vi "ExperimentCode_nodaq.vi"() -> ()   [LabVIEW 2017]
uses:
  <vilib>/Analysis/baseanly.llb/Mean (DBL).vi
  <vilib>/Instr/_visa.llb/VISA Configure Serial Port (Instr).vi
  <vilib>/express/express shared/transition.llb/Dynamic To Waveform Array.vi
  <vilib>/express/express signal manip/GetorSetDDTAttributes/Set DDT Attributes/SetT0.vi
  <vilib>/express/express shared/transition.llb/Waveform Array To Dynamic.vi
  <vilib>/express/express signal manip/GetorSetDDTAttributes/Set DDT Attributes/Set DDT Properties.xnode
  <vilib>/Analysis/NI_AALPro.lvlib
  <vilib>/Analysis/NI_AALBase.lvlib
panel:
  in  "Tab Control":enum32{"Setup ", "Experiment Controls", "Debug"}(tab)=enum."Experiment Controls"
  in  "Max Torque":dbl=21.3
  in  "Servo 1 Zero Offset":dbl
  in  "Servo 2 Zero Offset":dbl
  in  "Servo 3 Zero Offset":dbl
  in  "Servo 4 Zero Offset":dbl
  in  "Servo 5 Zero Offset":dbl
  in  "Servo 5 Torque Intercept":dbl
  in  "Servo 5 Torque Slope":dbl=1.0
  in  "Servo 5 Position Intercept":dbl
  in  "Servo 5 Position Slope":dbl=1.0
  in  "Servo 4 Torque Intercept":dbl
  in  "Servo 4 Torque Slope":dbl=1.0
  in  "Servo 4 Position Intercept":dbl
  in  "Servo 4 Position Slope":dbl=1.0
  in  "Servo 3 Torque Intercept":dbl
  in  "Servo 3 Torque Slope":dbl=1.0
  in  "Servo 3 Position Intercept":dbl
  in  "Servo 3 Position Slope":dbl=1.0
  in  "Servo 2 Torque Intercept":dbl
  in  "Servo 2 Torque Slope":dbl=1.0
  in  "Servo 2 Position Intercept":dbl
  in  "Servo 2 Position Slope":dbl=1.0
  in  "Servo 1 Torque Intercept":dbl
  in  "Servo 1 Torque Slope":dbl=1.0
  in  "Servo 1 Position Intercept":dbl
  in  "Servo 1 Position Slope":dbl=1.0
  in  "Plot Last x Seconds":dbl=10.0
  in  "COM Port":refnum<visa-resource-name>
  in  "Buad Rate":i32(ring)=115200 items=["2400"=2400, "4800"=4800, "9600"=9600, "14400"=14400, "19200"=19200, "28800"=28800, "38400"=38400, "57600"=57600, "115200"=115200]
  in  "Lowest Servo Angle":dbl=-65.0
  in  "Highest Servo Angle":dbl=65.0
  in  "Number of Servos":dbl=5.0
  out "Lift FFT":cluster{"timeout (s)":dbl, dbl, dbl[]}(graph)
  out "Maximum Torque Exceeded":bool
  in  "Amplitude (deg)":dbl=3.0
  in  "Save":bool
  in  "Stop VI":bool
  in  "Sample Frequency":dbl=100.0 step=50.0
  out "Servo Torque":cluster{" Time Offset":dbl, dbl, dbl[][]}(graph)
  in  "Amplitude (cm)":dbl=4.0
  in  "Length of Segments":dbl=10.0
  in  "Number of Waves":dbl=1.0
  in  "Wave Exponential":dbl=2.0
  in  "Frequency":dbl=1.0
  in  "Wave Form":u16(ring) items=["Sine", "Exponentional Sine", "Second Mode Bending", "Flat Plate"]
  in  "Wind Up Waveform":bool
  in  "Mode 1 Amplitude":dbl=0.1 step=0.1
  in  "Mode 2 Amplitude":dbl=0.2 step=0.1
  in  "Mode 1 Phase":dbl step=0.1
  in  "Mode 2 Phase":dbl=0.8499 step=0.1
  in  "Wind Down Waveform":bool
  in  "Wind Down Time":i32=5
  out "Waveform":cluster{"X Nodes":dbl[], "Y Nodes":dbl[]}[](graph)
  in  "Servo Input":bool
  in  "Send To Waveform to MBE":bool
  in  "Servo 5 Input":dbl
  in  "Servo 4 Input":dbl
  in  "Servo 3 Input":dbl
  in  "Servo 2 Input":dbl
  in  "Servo 1  Input":dbl
  out "Force and Moment Data":cluster{" Time Offset":dbl, "mean":dbl, dbl[][]}(graph)
  out "Minimum or Maximum Angle Exceeded":bool
  in  "Filename":path=path "test.tdms"
  in  "Comment":string
  out "Specified Time Delay":dbl
  out "Calculated Time Delay":dbl
  out "Time Elapsed":dbl
  out "Output Angles":dbl[](array[numeric])
  out "Input Angles":dbl[](array[numeric])
  out "Pos5 number":dbl
  out "Pos4 number":dbl
  out "Pos3 number":dbl
  out "Pos2 number":dbl
  out "Pos1 number":dbl
  out "Torq1 number":dbl
  out "Torq2 number":dbl
  out "Torq3 number":dbl
  out "Torq4 number":dbl
  out "Torq5 number":dbl
  out "Servo 1 Position":cluster{" Time Offset":dbl, "mean":dbl, dbl[][]}(graph)
  out "Servo 2 Position":cluster{" Time Offset":dbl, "mean":dbl, dbl[][]}(graph)
  out "Servo 3 Position":cluster{" Time Offset":dbl, "mean":dbl, dbl[][]}(graph)
  out "Servo 4 Position":cluster{" Time Offset":dbl, "mean":dbl, dbl[][]}(graph)
  out "Servo 5 Position":cluster{" Time Offset":dbl, "mean":dbl, dbl[][]}(graph)
  out "Sent to Arduino":string
  out "Bytes at port":cluster{i32, dbl, dbl[]}(graph)
  out "Read Buffer":string
  # "deg"
  # "deg"
  # "deg"
  # "deg"
  # "deg"
  # "Waveform"
  # "Manual"
  # "cm"
  # "Hz"
  # "Off"
  # "On"
  # "rad"
  # "rad"
  # "Off"
  # "On"
  # "Hz"
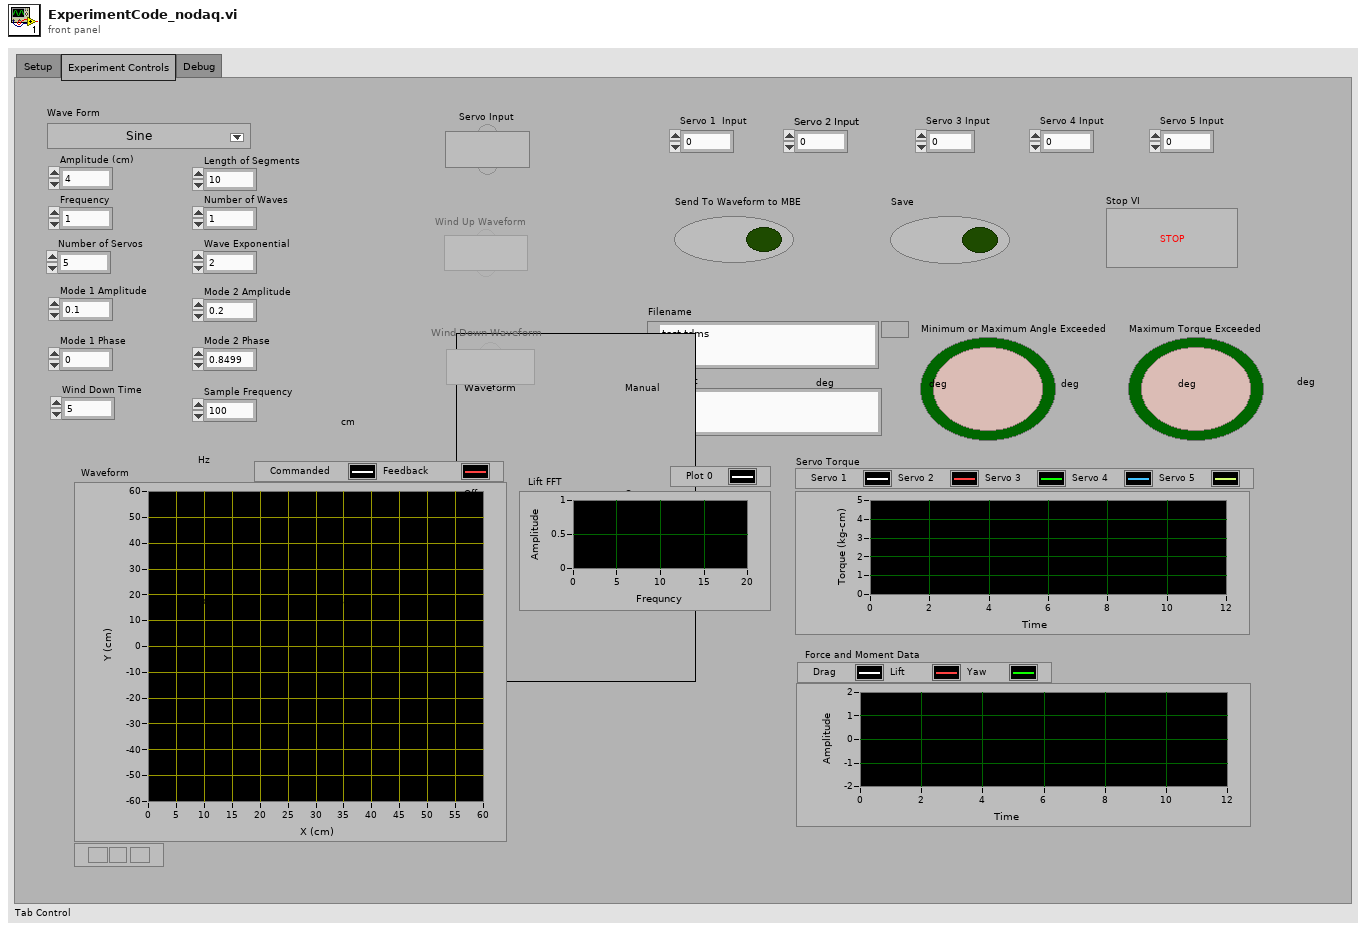
[diagram p1: front panel]
types:
  T1 = enum8{"Enabled", "Disabled", "Disabled and Grayed Out"}
  T2 = cluster{"Amplitude (deg)":dbl, "Amplitude (cm)":dbl, "Frequency":dbl, "Number of Waves":dbl, "Length of Segments":dbl, "Wave Exponential":dbl, "Number of Servos":dbl, "Mode 1 Amplitude":dbl, "Mode 2 Amplitude":dbl, "Mode 1 Phase":dbl, "Mode 2 Phase":dbl}
  T3 = cluster{"timeout (s)":dbl, "df":dbl, "Amp Spectrum Mag (Vrms)":dbl[]}
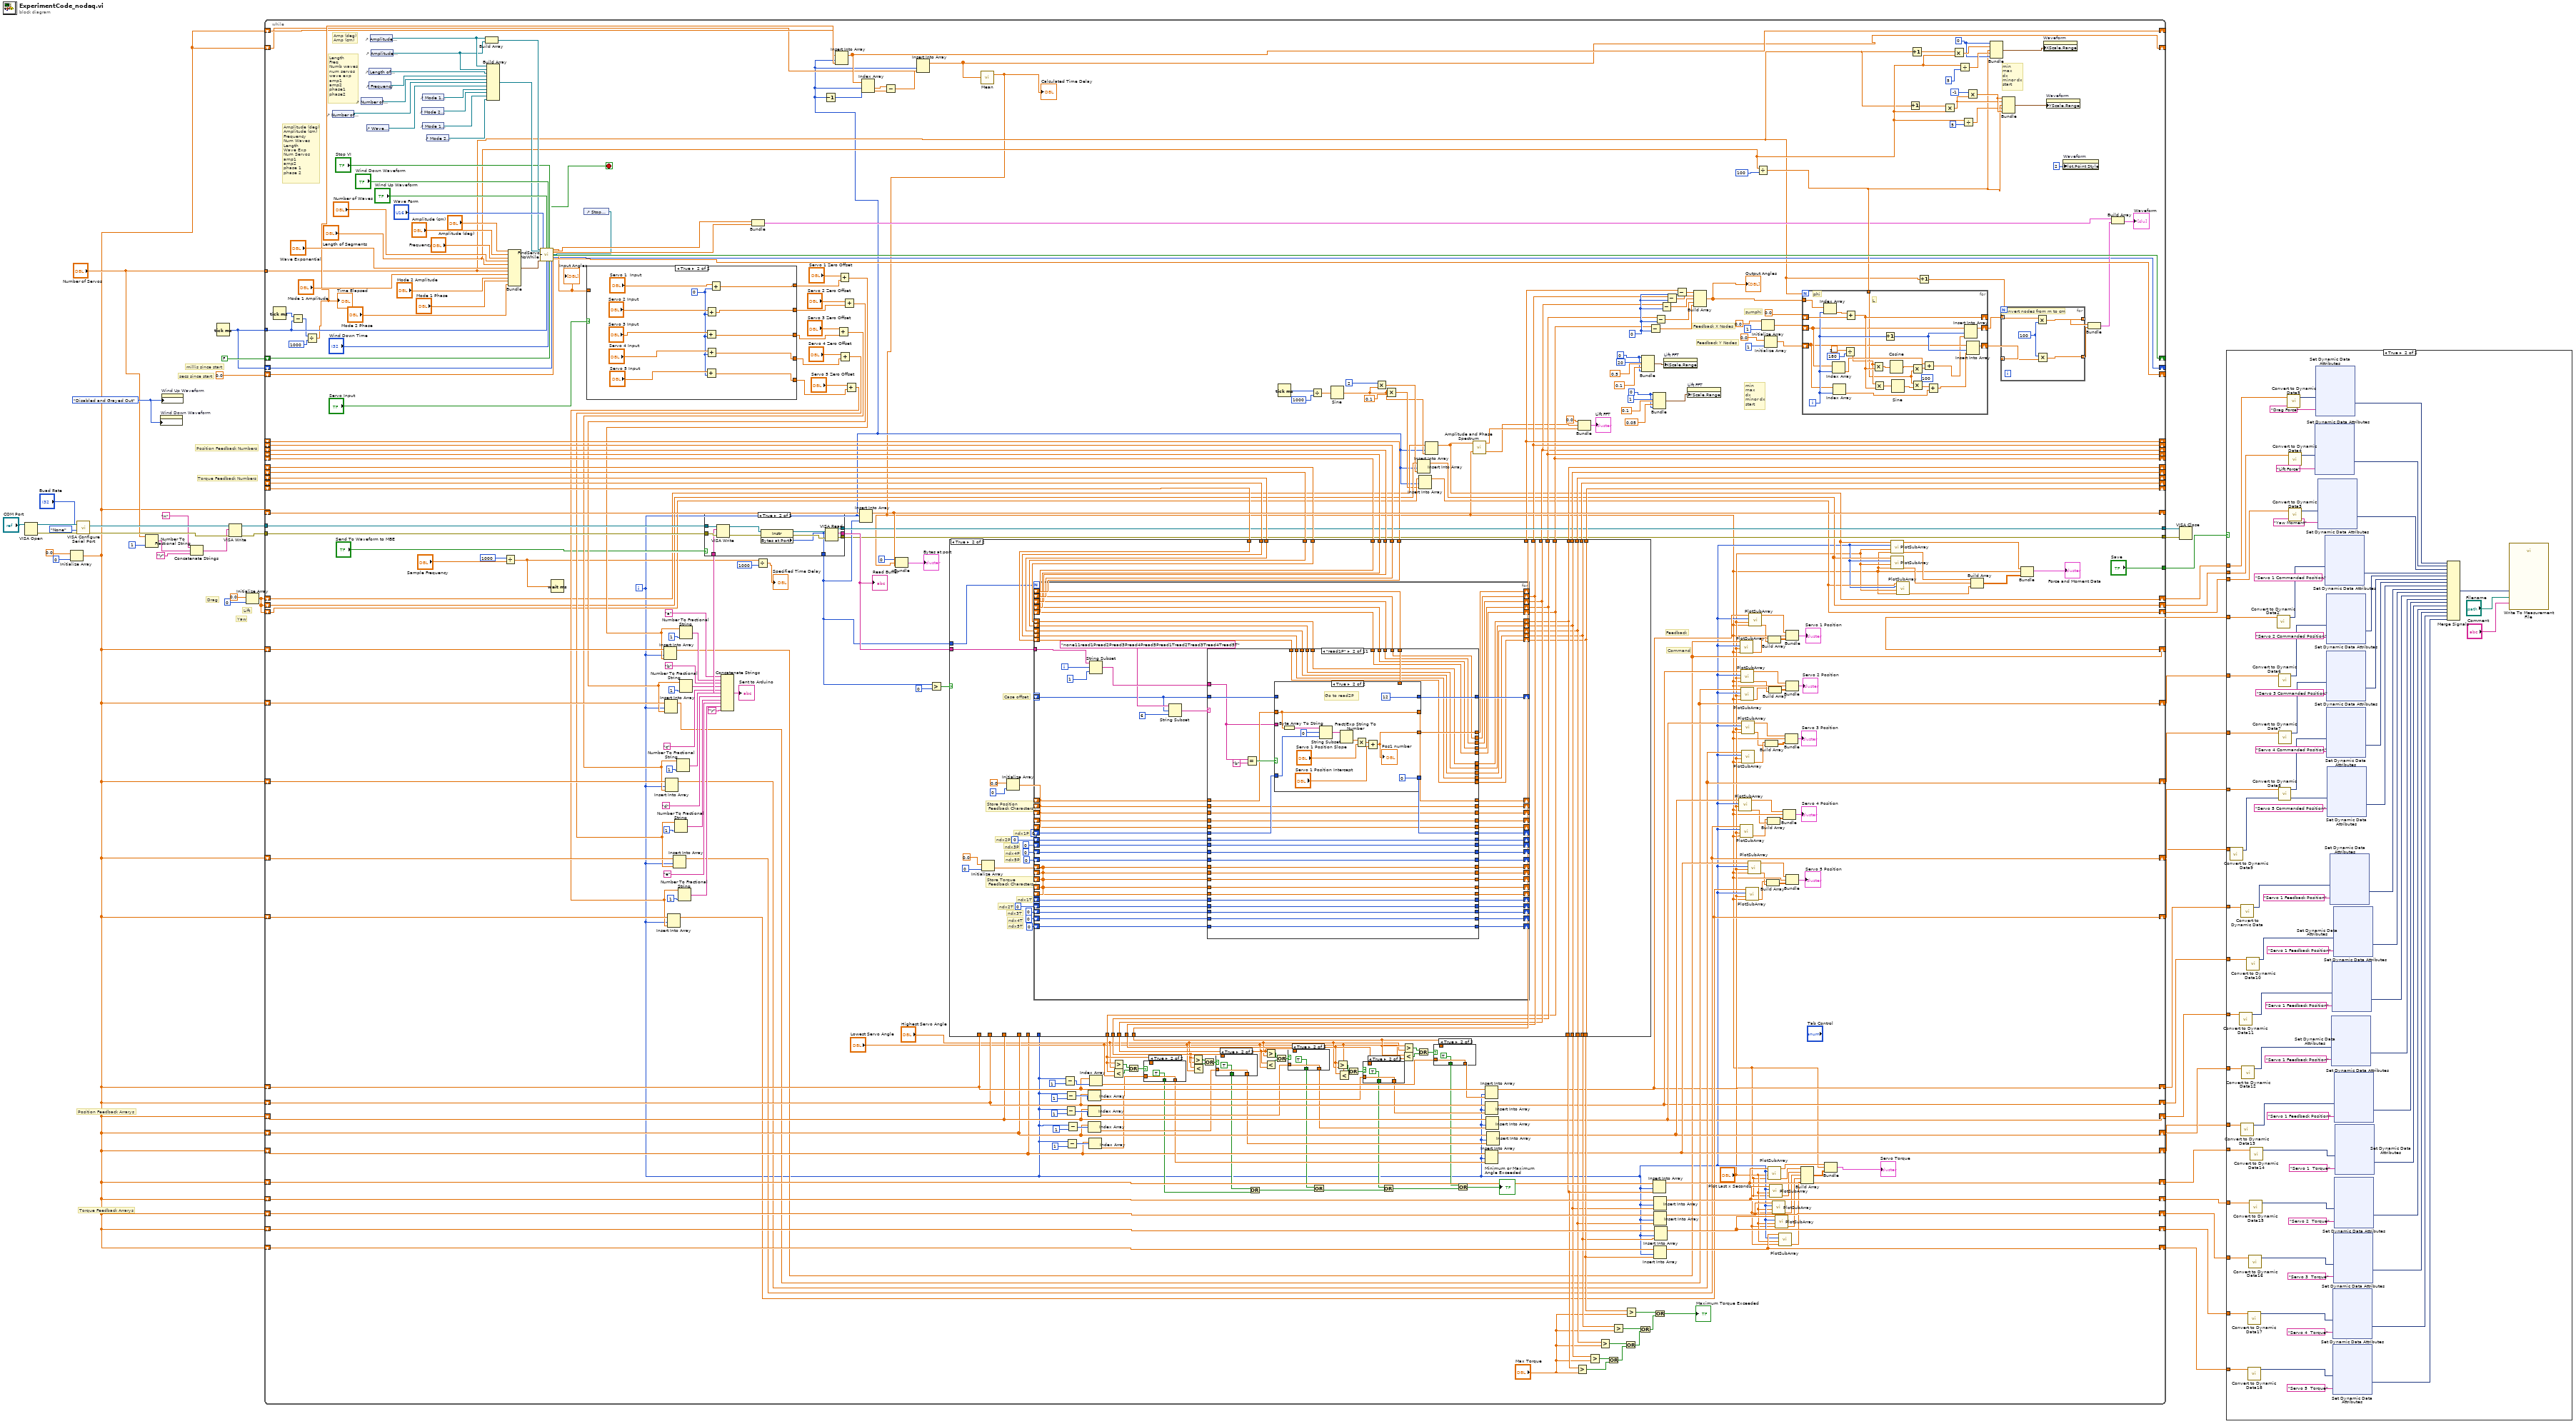
[diagram p0: block diagram]
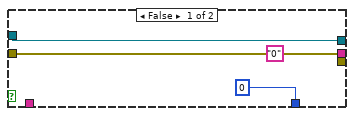
[diagram p3: hidden frame]
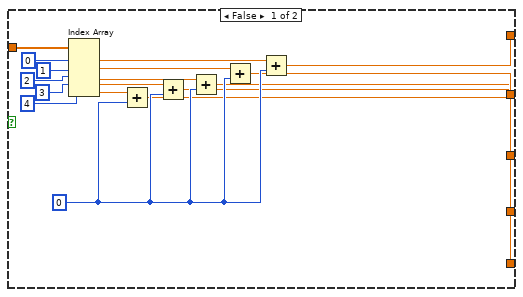
[diagram p4: hidden frame]
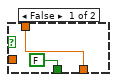
[diagram p5: hidden frame]
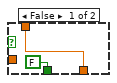
[diagram p6: hidden frame]
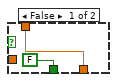
[diagram p7: hidden frame]
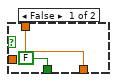
[diagram p8: hidden frame]
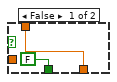
[diagram p9: hidden frame]
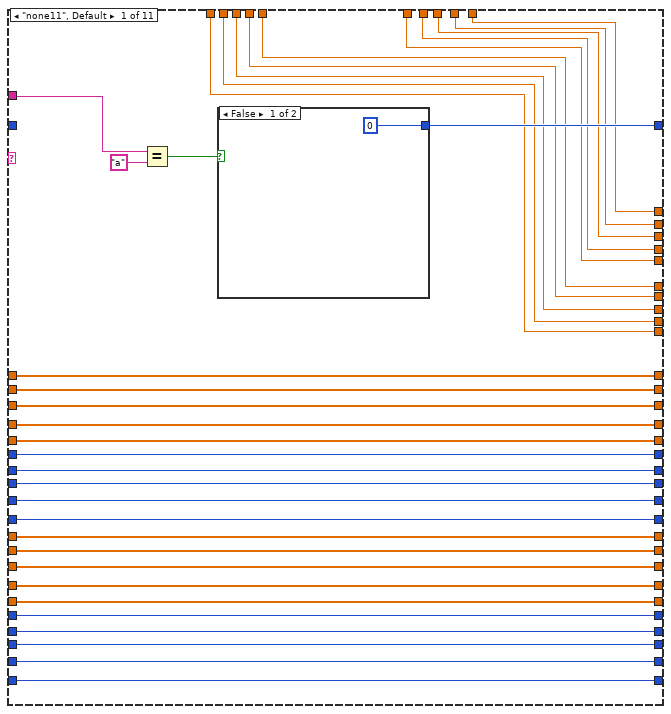
[diagram p11: hidden frame]
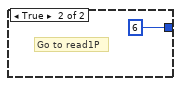
[diagram p12: hidden frame]
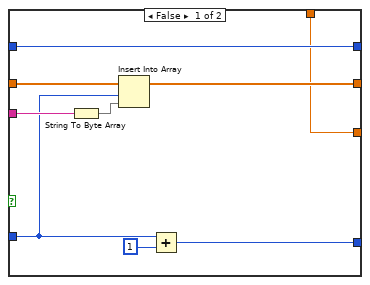
[diagram p13: hidden frame]
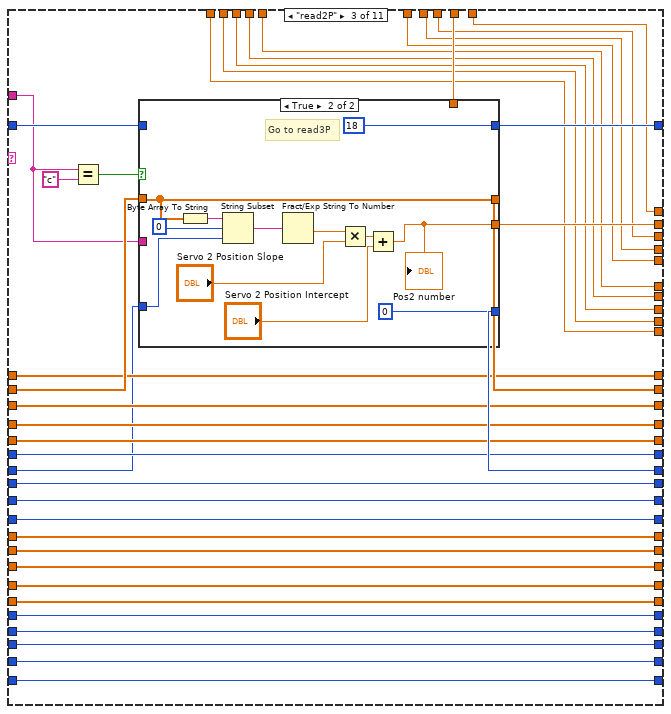
[diagram p14: hidden frame]
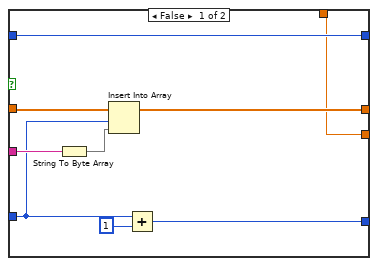
[diagram p15: hidden frame]
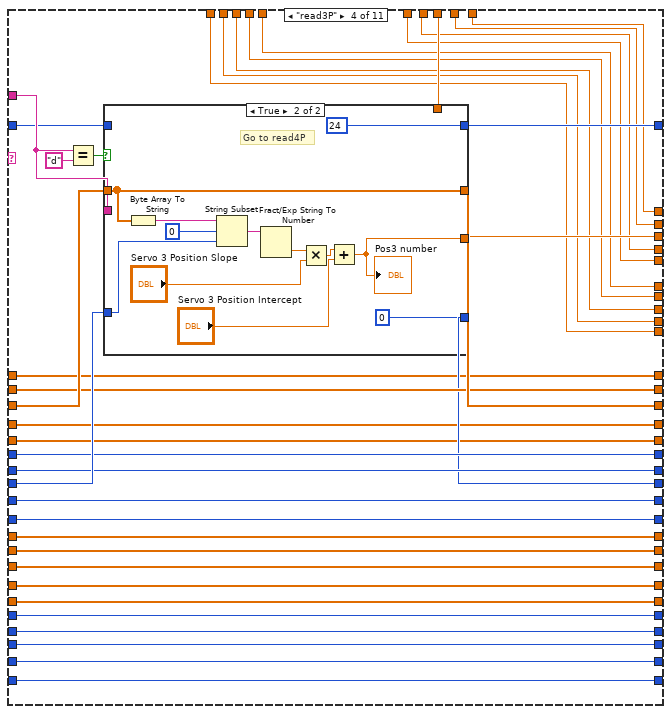
[diagram p16: hidden frame]
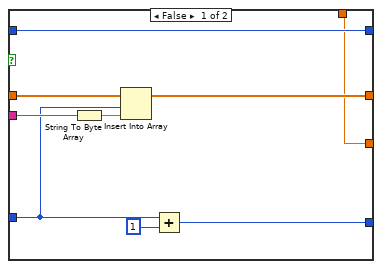
[diagram p17: hidden frame]
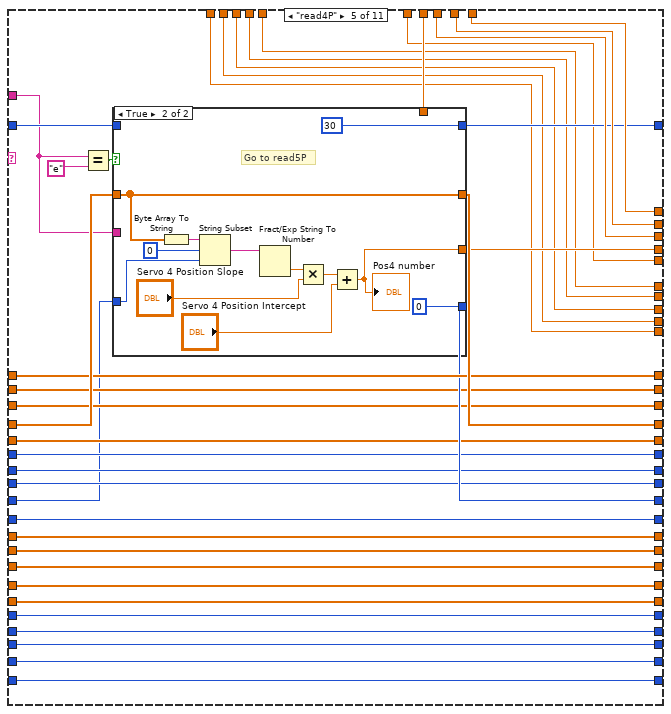
[diagram p18: hidden frame]
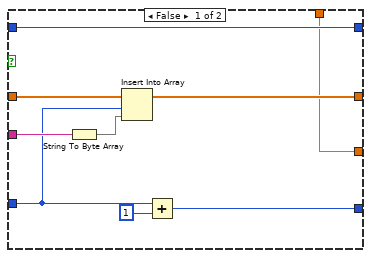
[diagram p19: hidden frame]
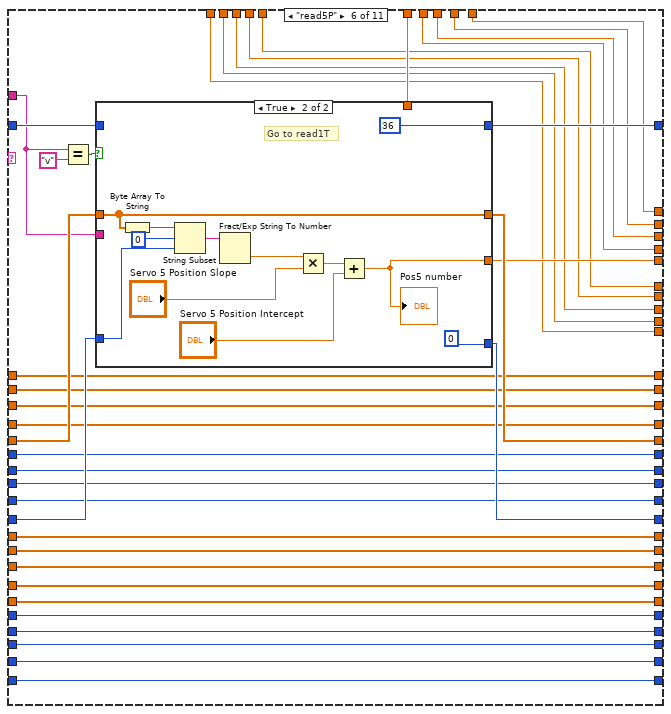
[diagram p20: hidden frame]
diagram:
  w28 = T1."Disabled and Grayed Out" ("Disabled")
  # "Yaw"
  # "Lift"
  # "secs since start"
  # "millis since start"
  # "Drag"
  # "Torque Feedback Numbers"
  # "Position Feedback Numbers"
  # "Torque Feedback Arrarys"
  # "Position Feedback Arrarys"
  n1 = VISA Open(VISA resource name="COM Port") -> (VISA resource name=w43:refnum<visa-resource-name>, error out=w41:errorcluster)  [unwired: 4 in]
  n2 = Initialize Array(0.0 ("element"), 0 ("dimension size")) -> (w1:dbl[])
  n3 = call-poly "VISA Configure Serial Port"("VISA resource name"=w43, "baud rate (9600)"="Buad Rate", "parity (0:none)"=enum16{"None", "Odd", "Even", "Mark", "Space"}."None", "error in (no error)"=w41) -> ("VISA resource name out"=w11:refnum<visa-resource-name>, "error out"=w10:errorcluster)  [unwired: 10 in]
  n4 = Number To Fractional String(number="Number of Servos", precision (6)=1) -> (F-format string=w6:string)  [unwired: 2 in]
  n5 = property on="Wind Down Waveform" class="Bool (strict)"("DisabledEnum"=w28) -> ()  [unwired: 2 in, 2 out]
  n6 = property on="Wind Up Waveform" class="Bool (strict)"("DisabledEnum"=w28) -> ()  [unwired: 2 in, 2 out]
  n7 = Concatenate Strings("n", w6, "\r") -> (w2:string)
  n8 = Tick Count (ms)() -> (millisecond timer value=w37:u32)
  n9 = VISA Write(VISA resource name=w11, write buffer=w2, error in (no error)=w10) -> (VISA resource name out=w9:refnum<visa-resource-name>, error out=w8:errorcluster)  [unwired: 1 out]
  n10 = Initialize Array(0.0 ("element"), 0 ("dimension size")) -> (w29:dbl[])
  n11 = while {
    shift-right: [w375] -> _
    shift-left: w1 -> [w376]
    shift-right: [w70] -> w35
    shift-left: w1 -> [w352]
    shift-right: [w72] -> w24
    shift-left: w1 -> [w351]
    shift-right: [w76] -> w23
    shift-left: w1 -> [w350]
    shift-right: [w78] -> w22
    shift-left: w1 -> [w349]
    shift-right: [w86] -> w21
    shift-left: w1 -> [w348]
    shift-right: [w69] -> w31
    shift-left: w1 -> [w316]
    shift-right: [w71] -> w20
    shift-left: w1 -> [w308]
    shift-right: [w75] -> w19
    shift-left: w1 -> [w305]
    shift-right: [w79] -> w18
    shift-left: w1 -> [w302]
    shift-right: [w85] -> w17
    shift-left: w1 -> [w272]
    shift-right: [w165] -> _
    shift-left: _ -> [w319]
    shift-right: [w164] -> _
    shift-left: _ -> [w338]
    shift-right: [w161] -> _
    shift-left: _ -> [w341]
    shift-right: [w163] -> _
    shift-left: _ -> [w340]
    shift-right: [w162] -> _
    shift-left: _ -> [w339]
    shift-right: [w332] -> _
    shift-left: _ -> [w333]
    shift-right: [w331] -> _
    shift-left: _ -> [w334]
    shift-right: [w330] -> _
    shift-left: _ -> [w335]
    shift-right: [w329] -> _
    shift-left: _ -> [w336]
    shift-right: [w328] -> _
    shift-left: _ -> [w337]
    shift-right: [w207] -> w16
    shift-left: w1 -> [w327]
    shift-right: [w205] -> w15
    shift-left: w1 -> [w326]
    shift-right: [w204] -> w14
    shift-left: w1 -> [w325]
    shift-right: [w203] -> w13
    shift-left: w1 -> [w324]
    shift-right: [w206] -> w12
    shift-left: w1 -> [w323]
    tunnel: w8 -> [w271]
    shift-right: [w66] -> w27
    shift-left: w29 -> [w127]
    tunnel: w37 -> [w103]
    shift-right: [w265] -> _
    shift-left: FALSE -> [w260]
    shift-right: [w93] -> _
    shift-left: w37 -> [w99]
    shift-right: [w264] -> _
    shift-left: 0.0 ("S since stop Shift Out") -> [w100]
    tunnel: ["Save"] -> w34
    tunnel: w9 -> [w270]
    tunnel: [w320] -> w33
    tunnel: [w134] -> w32
    shift-right: [w65] -> w26
    shift-left: w29 -> [w126]
    shift-right: [w64] -> w25
    shift-left: w29 -> [w125]
    shift-right: [w90] -> _
    shift-left: w1 -> [w97]
    tunnel: "Number of Servos" -> [w92]
    shift-right: [w87] -> _
    shift-left: w1 -> [w88]
    i -> [w59]
    stop <- w217 stop-if-true
    w109 = 0
    w113 = 0
    w150 = 0
    w166 = 0
    # "min\nmax\ndx\nminor dx\nstart"
    # "min\nmax\ndx\nminor dx\nstart"
    # "Feedback Y Nodes"
    # "Feedback X Nodes"
    # "sumphi"
    # "Command"
    # "Feedback"
    # "Amplitude (deg)\nAmplitude (cm)\nFrequency\nNum Waves\nLength\nWave Exp\nNum Servos\namp1\namp2\nphase 1\nphase 2"
    # "Amp (deg)\nAmp (cm)"
    # "Length\nFreq\nNumb waves\nnum servos\nwave exp\namp1\namp2\nphase1\nphase2"
    n12 = Tick Count (ms)() -> (millisecond timer value=w104:u32)
    n13 = Subtract(x=w104, y=w103) -> (x-y=w102:u32)
    n14 = Divide(x=w102, y=1000) -> (x/y=w98:dbl)
    "Time Elapsed" <- w98
    n15 = control-ref of="Number of Servos"() -> (w91:refnum<vi>)
    n16 = control-ref of="Number of Waves"() -> (w240:refnum<vi>)
    n17 = control-ref of="Wave Exponential"() -> (w239:refnum<vi>)
    n18 = control-ref of="Length of Segments"() -> (w242:refnum<vi>)
    n19 = control-ref of="Frequency"() -> (w241:refnum<vi>)
    n20 = control-ref of="Amplitude (deg)"() -> (w222:refnum<vi>)
    n21 = control-ref of="Amplitude (cm)"() -> (w221:refnum<vi>)
    n22 = control-ref of="Mode 2 Amplitude"() -> (w237:refnum<vi>)
    n23 = control-ref of="Mode 1 Amplitude"() -> (w238:refnum<vi>)
    n24 = control-ref of="Mode 1 Phase"() -> (w236:refnum<vi>)
    n25 = control-ref of="Mode 2 Phase"() -> (w235:refnum<vi>)
    n26 = Build Array(w222, w221) -> (w224:refnum<vi>[])
    n27 = Build Array(w222, w221, w242, w241, w240, w91, w239, w238, w237, w236, w235) -> (w223:refnum<vi>[])
    n28 = Divide(x=1000, y="Sample Frequency") -> (x/y=w106:dbl)
    n29 = Bundle("Amplitude (deg)"="Amplitude (deg)", "Amplitude (cm)"="Amplitude (cm)", "Frequency"="Frequency", "Number of Waves"="Number of Waves", "Length of Segments"="Length of Segments", "Wave Exponential"="Wave Exponential", "Number of Servos"=w92, "Mode 1 Amplitude"="Mode 1 Amplitude", "Mode 2 Amplitude"="Mode 2 Amplitude", "Mode 1 Phase"="Mode 1 Phase", "Mode 2 Phase"="Mode 2 Phase") -> (w225:T2)  [unwired: 1 in]
    n30 = Wait (ms)(milliseconds to wait=w106) -> ()  [unwired: 1 out]
    n31 = control-ref of="Stop Reference"() -> (w259:refnum<vi>)
    n32 = call "FindServo_NoWhile.vi"("Amplitude Reference Array"=w224, "Parameter Reference Arrary"=w223, "Parameter Cluster"=w225, "Wave Form"="Wave Form", "Wind Up"="Wind Up Waveform", "Start Time (Tick Count-millis)"=w103, "Wind Down"="Wind Down Waveform", "Wind Down Time"="Wind Down Time", "Stop In"="Stop VI", "Stop Pressed Shift In (False)"=w260, "Ms Since Stop Shift In (Start Time)"=w99, "Stop In Reference"=w259, "S since stop Shift In"=w100) -> ("Stop Out"=w217:bool, "phi"=w135:dbl[], "X Nodes"=w263:dbl[], "Y Nodes"=w262:dbl[], "Stop Pressed Shift Out (False)"=w265:bool, "MS Since Stop Shift Out"=w93:u32, "S since stop Shift Out"=w264:dbl)  [unwired: 8 in]
    "Input Angles" <- w135
    n33 = case shown="True" "Servo Input" {
      tunnel: [w425 w448] -> w253
      tunnel: [w424 w440] -> w252
      tunnel: [w423 w439] -> w251
      tunnel: [w422 w444] -> w250
      tunnel: [w421 w445] -> w249
      tunnel: w135 -> [w437 _]
      frame False {
        w426 = 0
        n34 = Index Array(array=w437, index #1=0, index #2=1, index #3=2, index #4=3, index #5=4) -> (element #1=w431:dbl, element #2=w430:dbl, element #3=w429:dbl, element #4=w428:dbl, element #5=w427:dbl)
        n35 = Add(x=w427, y=w426) -> (x+y=w421:dbl)
        n36 = Add(x=w428, y=w426) -> (x+y=w422:dbl)
        n37 = Add(x=w429, y=w426) -> (x+y=w423:dbl)
        n38 = Add(x=w430, y=w426) -> (x+y=w424:dbl)
        n39 = Add(x=w431, y=w426) -> (x+y=w425:dbl)
      }
      frame True {
        w438 = 0
        n40 = Add(x="Servo 3 Input", y=w438) -> (x+y=w439:dbl)
        n41 = Add(x="Servo 5 Input", y=w438) -> (x+y=w445:dbl)
        n42 = Add(x="Servo 2 Input", y=w438) -> (x+y=w440:dbl)
        n43 = Add(x="Servo 4 Input", y=w438) -> (x+y=w444:dbl)
        n44 = Add(x="Servo 1  Input", y=w438) -> (x+y=w448:dbl)
      }
    }
    n45 = Bundle("X Nodes"=w263, "Y Nodes"=w262) -> (w145:cluster{"X Nodes":dbl[], "Y Nodes":dbl[]})  [unwired: 1 in]
    n46 = Divide(x=w106, y=1000) -> (x/y=→"Specified Time Delay":dbl)
    n47 = Decrement(x=w59) -> (x-1=w94:i32)
    n48 = Insert Into Array(array=w97, index=w59, new element=w98) -> (w90:dbl[])
    n49 = Add(x="Servo 3 Zero Offset", y=w251) -> (x+y=w246:dbl)
    n50 = Insert Into Array(array=w350, index=w59, new element=w246) -> (w76:dbl[])
    n51 = Number To Fractional String(number=w246, precision (6)=1) -> (F-format string=w371:string)  [unwired: 2 in]
    n52 = Add(x="Servo 1 Zero Offset", y=w253) -> (x+y=w244:dbl)
    n53 = Insert Into Array(array=w352, index=w59, new element=w244) -> (w70:dbl[])
    n54 = Number To Fractional String(number=w244, precision (6)=1) -> (F-format string=w373:string)  [unwired: 2 in]
    n55 = Add(x="Servo 4 Zero Offset", y=w250) -> (x+y=w247:dbl)
    n56 = Insert Into Array(array=w349, index=w59, new element=w247) -> (w78:dbl[])
    n57 = Number To Fractional String(number=w247, precision (6)=1) -> (F-format string=w364:string)  [unwired: 2 in]
    n58 = Add(x="Servo 2 Zero Offset", y=w252) -> (x+y=w245:dbl)
    n59 = Insert Into Array(array=w351, index=w59, new element=w245) -> (w72:dbl[])
    n60 = Number To Fractional String(number=w245, precision (6)=1) -> (F-format string=w372:string)  [unwired: 2 in]
    n61 = Add(x="Servo 5 Zero Offset", y=w249) -> (x+y=w248:dbl)
    n62 = Insert Into Array(array=w348, index=w59, new element=w248) -> (w86:dbl[])
    n63 = Number To Fractional String(number=w248, precision (6)=1) -> (F-format string=w363:string)  [unwired: 2 in]
    n64 = Concatenate Strings("a", w373, "b", w372, "c", w371, "d", w364, "e", w363, "\r") -> (w374:string)
    "Sent to Arduino" <- w374
    n65 = case shown="True" "Send To Waveform to MBE" {
      tunnel: w374 -> [_ w410]
      tunnel: ["0" w420] -> w359
      tunnel: [w408 w419] -> w134
      tunnel: [w409 w418] -> w320
      tunnel: [0 w413] -> w220
      tunnel: w271 -> [w408 w412]
      tunnel: w270 -> [w409 w411]
      frame False {
      }
      frame True {
        n66 = VISA Write(VISA resource name=w411, write buffer=w410, error in (no error)=w412) -> (VISA resource name out=w417:refnum<visa-resource-name>, error out=w414:errorcluster)  [unwired: 1 out]
        n67 = property class="Instr"(reference=w417, error in=w414) -> (reference out=w416:refnum<visa-resource-name>, error out=w415:errorcluster, "Bytes at Port"=w413:u32)
        n68 = VISA Read(VISA resource name=w416, byte count=w413, error in (no error)=w415) -> (VISA resource name out=w418:refnum<visa-resource-name>, read buffer=w420:string, error out=w419:errorcluster)  [unwired: 1 out]
      }
    }
    "Read Buffer" <- w359
    n69 = Insert Into Array(array=w376, index=w59, new element=w220) -> (w375:dbl[])
    n70 = Index Array(array=w90, index #1=w59, index #2=w94) -> (element #1=w96:dbl, element #2=w95:dbl)
    n71 = Subtract(x=w96, y=w95) -> (x-y=w89:dbl)
    n72 = Insert Into Array(array=w88, index=w59, new element=w89) -> (w87:dbl[])
    n73 = Greater?(x=w220, y=0) -> (0:w322:bool)
    n74 = case shown="True" w322 {
      tunnel: w220 -> [_ w479]
      tunnel: w359 -> [_ w517]
      tunnel: [w478 w491] -> w311
      tunnel: w59 -> [_ _]
      tunnel: w316 -> [_ _]
      tunnel: [w477 w490] -> w293
      tunnel: [w476 w489] -> w287
      tunnel: [w475 w488] -> w281
      tunnel: [w474 w487] -> w277
      tunnel: w308 -> [_ _]
      tunnel: w305 -> [_ _]
      tunnel: w302 -> [_ _]
      tunnel: w272 -> [_ _]
      tunnel: w319 -> [w478 w508]
      tunnel: w338 -> [w477 w507]
      tunnel: w341 -> [w476 w506]
      tunnel: w340 -> [w475 w505]
      tunnel: w339 -> [w474 w504]
      tunnel: [w478 w491] -> w165
      tunnel: [w477 w490] -> w164
      tunnel: [w476 w489] -> w161
      tunnel: [w475 w488] -> w163
      tunnel: [w474 w487] -> w162
      tunnel: w337 -> [w469 w481]
      tunnel: w336 -> [w470 w483]
      tunnel: w335 -> [w471 w503]
      tunnel: w334 -> [w472 w502]
      tunnel: w333 -> [w473 w501]
      tunnel: [w473 w486] -> w332
      tunnel: [w472 w485] -> w331
      tunnel: [w471 w484] -> w330
      tunnel: [w470 w482] -> w329
      tunnel: [w469 w480] -> w328
      tunnel: [w473 w486] -> w194
      tunnel: [w472 w485] -> w190
      tunnel: [w471 w484] -> w191
      tunnel: [w470 w482] -> w192
      tunnel: [w469 w480] -> w193
      frame False {
      }
      frame True {
        # "Store Torque\n Feedback Characters"
        # "ndx5T"
        # "ndx4T"
        # "ndx3T"
        # "ndx2T"
        # "ndx1T"
        # "Store Position\n Feedback Characters"
        # "ndx5P"
        # "ndx4P"
        # "ndx3P"
        # "ndx2P"
        # "ndx1P"
        # "Case offset"
        n75 = Initialize Array(0.0 ("element"), 0 ("dimension size")) -> (w498:dbl[])
        n76 = Initialize Array(0.0 ("element"), 0 ("dimension size")) -> (w511:dbl[])
        n77 = for {
          N: w479 -> [_]
          tunnel: w517 -> [w585]
          shift-right: [w583] -> _
          shift-left: 1 -> [w528]
          shift-right: [w582] -> _
          shift-left: 0 -> [w581]
          shift-right: [w579] -> _
          shift-left: w511 -> [w580]
          shift-right: [w577] -> _
          shift-left: w511 -> [w578]
          shift-right: [w573] -> _
          shift-left: 0 -> [w576]
          shift-right: [w574] -> _
          shift-left: 0 -> [w575]
          shift-right: [w571] -> _
          shift-left: w511 -> [w572]
          shift-right: [w563] -> _
          shift-left: w511 -> [w570]
          shift-right: [w564] -> _
          shift-left: w511 -> [w569]
          shift-right: [w567] -> _
          shift-left: 0 -> [w568]
          shift-right: [w565] -> _
          shift-left: 0 -> [w566]
          shift-right: [w550] -> _
          shift-left: w498 -> [w551]
          shift-right: [w549] -> _
          shift-left: w498 -> [w548]
          shift-right: [w547] -> _
          shift-left: w498 -> [w546]
          shift-right: [w545] -> _
          shift-left: w498 -> [w544]
          shift-right: [w543] -> _
          shift-left: w498 -> [w542]
          shift-right: [w541] -> _
          shift-left: 0 -> [w540]
          shift-right: [w539] -> _
          shift-left: 0 -> [w538]
          shift-right: [w537] -> _
          shift-left: 0 -> [w536]
          shift-right: [w534] -> _
          shift-left: 0 -> [w535]
          shift-right: [w533] -> _
          shift-left: 0 -> [w532]
          shift-right: [w527] -> w491
          shift-left: w508 -> [w558]
          shift-right: [w526] -> w490
          shift-left: w507 -> [w562]
          shift-right: [w525] -> w489
          shift-left: w506 -> [w561]
          shift-right: [w524] -> w488
          shift-left: w505 -> [w560]
          shift-right: [w523] -> w487
          shift-left: w504 -> [w559]
          shift-right: [w522] -> w486
          shift-left: w501 -> [w552]
          shift-right: [w521] -> w485
          shift-left: w502 -> [w553]
          shift-right: [w520] -> w484
          shift-left: w503 -> [w554]
          shift-right: [w519] -> w482
          shift-left: w483 -> [w555]
          shift-right: [w518] -> w480
          shift-left: w481 -> [w556]
          i -> [w529]
          n78 = String Subset(string=w585, offset (0)=w529, length (rest)=1 ("length (rest)")) -> (substring=w557:string)
          n79 = String Subset(string="none11read1Pread2Pread3Pread4Pread5Pread1Tread2Tread3Tread4Tread5T", offset (0)=w528, length (rest)=6 ("length (rest)")) -> (substring=w531:string)
          n80 = case shown="\"read1P\"" w531 {
            tunnel: w557 -> [w620 w654 w710 w764 w831 w890 w951 w1010 w1069 w1128 w1187]
            tunnel: [w617 w657 w712 w771 w817 w893 w954 w1013 w1072 w1131 w1190] -> w583
            tunnel: [w616 w652 w714 w776 w829 w883 w946 w1005 w1064 w1123 w1182] -> w582
            tunnel: w581 -> [w616 w653 w714 w776 w829 w883 w946 w1005 w1064 w1123 w1182]
            tunnel: w580 -> [w613 w655 w709 w759 w835 w887 w950 w1009 w1068 w1127 w1186]
            tunnel: [w613 w658 w709 w759 w835 w887 w950 w1009 w1068 w1127 w1186] -> w579
            tunnel: w578 -> [w614 w651 w719 w772 w827 w886 w949 w1008 w1067 w1126 w1185]
            tunnel: [w614 w651 w718 w772 w827 w886 w949 w1008 w1067 w1126 w1185] -> w577
            tunnel: w576 -> [w615 w647 w697 w775 w828 w882 w945 w1004 w1063 w1122 w1181]
            tunnel: [w615 w647 w717 w775 w828 w882 w945 w1004 w1063 w1122 w1181] -> w573
            tunnel: w528 -> [_ w656 w713 w756 w832 w892 w953 w1012 w1071 w1130 w1189]
            tunnel: w575 -> [w610 w646 w711 w777 w824 w881 w944 w1003 w1062 w1121 w1180]
            tunnel: [w610 w646 w711 w768 w824 w881 w944 w1003 w1062 w1121 w1180] -> w574
            tunnel: w572 -> [w607 w650 w708 w774 w826 w885 w948 w1007 w1066 w1125 w1184]
            tunnel: [w607 w650 w708 w773 w826 w885 w948 w1007 w1066 w1125 w1184] -> w571
            tunnel: w570 -> [w608 w649 w707 w767 w837 w884 w947 w1006 w1065 w1124 w1183]
            tunnel: w569 -> [w609 w648 w706 w766 w825 w895 w938 w997 w1049 w1108 w1167]
            tunnel: w568 -> [w612 w645 w705 w770 w816 w880 w943 w1002 w1061 w1120 w1179]
            tunnel: [w612 w645 w705 w770 w830 w880 w943 w1002 w1061 w1120 w1179] -> w567
            tunnel: w566 -> [w611 w644 w704 w769 w823 w889 w935 w986 w1046 w1102 w1164]
            tunnel: [w611 w644 w704 w769 w823 w888 w935 w986 w1046 w1102 w1164] -> w565
            tunnel: [w609 w648 w706 w766 w825 w894 w938 w997 w1049 w1108 w1167] -> w564
            tunnel: [w608 w649 w707 w767 w836 w884 w947 w1006 w1065 w1124 w1183] -> w563
            tunnel: [w602 w643 w701 w757 w818 w879 w942 w1001 w1060 w1119 w1178] -> w527
            tunnel: w558 -> [w602 w642 w701 w757 w818 w879 w942 w1001 w1060 w1119 w1178]
            tunnel: [w606 w641 w703 w763 w822 w874 w939 w998 w1057 w1116 w1175] -> w526
            tunnel: w562 -> [w606 w641 w702 w763 w822 w874 w939 w998 w1057 w1116 w1175]
            tunnel: [w605 w640 w698 w762 w819 w877 w941 w1000 w1059 w1118 w1177] -> w525
            tunnel: w561 -> [w605 w640 w698 w761 w819 w877 w941 w1000 w1059 w1118 w1177]
            tunnel: [w604 w639 w700 w760 w821 w875 w940 w999 w1058 w1117 w1176] -> w524
            tunnel: w560 -> [w604 w639 w700 w760 w820 w875 w940 w999 w1058 w1117 w1176]
            tunnel: [w603 w638 w699 w758 w800 w878 w931 w981 w1055 w1115 w1174] -> w523
            tunnel: w559 -> [w603 w638 w699 w758 w800 w876 w931 w981 w1055 w1115 w1174]
            tunnel: w556 -> [w597 w633 w692 w751 w811 w869 w919 w977 w1050 w1109 w1173]
            tunnel: w555 -> [w598 w634 w693 w752 w812 w870 w920 w978 w1052 w1114 w1168]
            tunnel: w554 -> [w599 w635 w694 w753 w813 w871 w921 w979 w1056 w1111 w1169]
            tunnel: w553 -> [w600 w636 w695 w754 w814 w872 w922 w983 w1053 w1112 w1170]
            tunnel: w552 -> [w601 w637 w696 w755 w815 w873 w932 w982 w1054 w1113 w1171]
            tunnel: [w601 w637 w696 w755 w815 w873 w930 w982 w1054 w1113 w1171] -> w522
            tunnel: [w600 w636 w695 w754 w814 w872 w922 w980 w1053 w1112 w1170] -> w521
            tunnel: [w599 w635 w694 w753 w813 w871 w921 w979 w1051 w1111 w1169] -> w520
            tunnel: [w598 w634 w693 w752 w812 w870 w920 w978 w1052 w1110 w1168] -> w519
            tunnel: [w597 w633 w692 w751 w811 w869 w919 w977 w1050 w1109 w1172] -> w518
            tunnel: w551 -> [w596 w632 w691 w750 w810 w868 w937 w994 w1043 w1105 w1154]
            tunnel: [w596 w632 w691 w750 w810 w868 w936 w994 w1043 w1105 w1154] -> w550
            tunnel: [w595 w631 w690 w749 w809 w867 w929 w995 w1042 w1104 w1155] -> w549
            tunnel: w548 -> [w595 w631 w690 w749 w809 w867 w929 w996 w1042 w1104 w1155]
            tunnel: [w594 w630 w689 w748 w808 w866 w928 w993 w1047 w1103 w1156] -> w547
            tunnel: w546 -> [w594 w630 w689 w748 w808 w866 w928 w993 w1048 w1103 w1156]
            tunnel: [w593 w629 w688 w747 w807 w865 w927 w992 w1041 w1107 w1157] -> w545
            tunnel: w544 -> [w593 w629 w688 w747 w807 w865 w927 w992 w1041 w1106 w1157]
            tunnel: [w592 w628 w687 w746 w806 w864 w926 w991 w1040 w1098 w1166] -> w543
            tunnel: w542 -> [w592 w628 w687 w746 w806 w864 w926 w991 w1040 w1098 w1165]
            tunnel: [w591 w627 w686 w745 w805 w863 w933 w990 w1039 w1099 w1158] -> w541
            tunnel: w540 -> [w591 w627 w686 w745 w805 w863 w934 w990 w1039 w1099 w1158]
            tunnel: [w590 w626 w685 w744 w804 w862 w925 w985 w1038 w1097 w1159] -> w539
            tunnel: w538 -> [w590 w626 w685 w744 w804 w862 w925 w984 w1038 w1097 w1159]
            tunnel: [w589 w625 w684 w743 w803 w861 w924 w989 w1045 w1096 w1160] -> w537
            tunnel: w536 -> [w589 w625 w684 w743 w803 w861 w924 w989 w1044 w1096 w1160]
            tunnel: w535 -> [w588 w624 w683 w742 w802 w860 w923 w988 w1037 w1100 w1161]
            tunnel: [w588 w624 w683 w742 w802 w860 w923 w988 w1037 w1101 w1161] -> w534
            tunnel: [w587 w623 w682 w741 w801 w859 w918 w987 w1036 w1095 w1163] -> w533
            tunnel: w532 -> [w587 w623 w682 w741 w801 w859 w918 w987 w1036 w1095 w1162]
            frame "none11", Default {
              n81 = Equal?(x=w620, y="a") -> (x = y?=w618:bool)
              n82 = case shown="False" w618 {
                tunnel: [0 6] -> w617
                frame False {
                }
                frame True {
                  # "Go to read1P"
                }
              }
            }
            frame "read1P" {
              n83 = Equal?(x=w654, y="b") -> (x = y?=w659:bool)
              n84 = case shown="True" w659 {
                tunnel: [w669 0] -> w652
                tunnel: w655 -> [w663 w677]
                tunnel: [w667 w677] -> w658
                tunnel: w654 -> [w666 _]
                tunnel: [w664 12] -> w657
                tunnel: w656 -> [w664 _]
                tunnel: w653 -> [w662 w676]
                tunnel: [w661 w674] -> w643
                tunnel: w642 -> [w661 _]
                frame False {
                  n85 = String To Byte Array(string=w666) -> (unsigned byte array=w665:u8[])
                  n86 = Insert Into Array(array=w663, index=w662, new element=w665) -> (w667:dbl[])
                  n87 = Add(x=w662, y=1) -> (x+y=w669:i32)
                }
                frame True {
                  # "Go to read2P"
                  n88 = Byte Array To String(unsigned byte array=w677) -> (string=w678:string)
                  n89 = String Subset(string=w678, offset (0)=0, length (rest)=w676) -> (substring=w675:string)
                  n90 = Fract/Exp String To Number(string=w675) -> (number=w673:dbl)  [unwired: 3 in, 1 out]
                  n91 = Multiply(x=w673, y="Servo 1 Position Slope") -> (x*y=w672:dbl)
                  n92 = Add(x=w672, y="Servo 1 Position Intercept") -> (x+y=w674:dbl)
                  "Pos1 number" <- w674
                }
              }
            }
            frame "read2P" {
              n93 = Equal?(x=w710, y="c") -> (x = y?=w715:bool)
              n94 = case shown="True" w715 {
                tunnel: [w728 0] -> w717
                tunnel: w697 -> [w722 w737]
                tunnel: w719 -> [w726 w735]
                tunnel: [w725 w735] -> w718
                tunnel: w710 -> [w724 _]
                tunnel: [w721 18] -> w712
                tunnel: w713 -> [w721 _]
                tunnel: [w720 w731] -> w703
                tunnel: w702 -> [w720 _]
                frame False {
                  n95 = String To Byte Array(string=w724) -> (unsigned byte array=w723:u8[])
                  n96 = Insert Into Array(array=w726, index=w722, new element=w723) -> (w725:dbl[])
                  n97 = Add(x=w722, y=1) -> (x+y=w728:i32)
                }
                frame True {
                  # "Go to read3P"
                  n98 = Byte Array To String(unsigned byte array=w735) -> (string=w734:string)
                  n99 = String Subset(string=w734, offset (0)=0, length (rest)=w737) -> (substring=w736:string)
                  n100 = Fract/Exp String To Number(string=w736) -> (number=w732:dbl)  [unwired: 3 in, 1 out]
                  n101 = Multiply(x=w732, y="Servo 2 Position Slope") -> (x*y=w733:dbl)
                  n102 = Add(x=w733, y="Servo 2 Position Intercept") -> (x+y=w731:dbl)
                  "Pos2 number" <- w731
                }
              }
            }
            frame "read3P" {
              n103 = Equal?(x=w764, y="d") -> (x = y?=w778:bool)
              n104 = case shown="True" w778 {
                tunnel: [w787 0] -> w768
                tunnel: w777 -> [w781 w794]
                tunnel: w774 -> [w785 w795]
                tunnel: [w784 w795] -> w773
                tunnel: w764 -> [w783 _]
                tunnel: [w780 24] -> w771
                tunnel: w756 -> [w780 _]
                tunnel: [w779 w788] -> w762
                tunnel: w761 -> [w779 _]
                frame False {
                  n105 = String To Byte Array(string=w783) -> (unsigned byte array=w782:u8[])
                  n106 = Insert Into Array(array=w785, index=w781, new element=w782) -> (w784:dbl[])
                  n107 = Add(x=w781, y=1) -> (x+y=w787:i32)
                }
                frame True {
                  # "Go to read4P"
                  n108 = Byte Array To String(unsigned byte array=w795) -> (string=w796:string)
                  n109 = String Subset(string=w796, offset (0)=0, length (rest)=w794) -> (substring=w793:string)
                  n110 = Fract/Exp String To Number(string=w793) -> (number=w791:dbl)  [unwired: 3 in, 1 out]
                  n111 = Multiply(x=w791, y="Servo 3 Position Slope") -> (x*y=w792:dbl)
                  n112 = Add(x=w792, y="Servo 3 Position Intercept") -> (x+y=w788:dbl)
                  "Pos3 number" <- w788
                }
              }
            }
            frame "read4P" {
              n113 = Equal?(x=w831, y="e") -> (x = y?=w833:bool)
              n114 = case shown="True" w833 {
                tunnel: [w846 0] -> w830
                tunnel: w816 -> [w840 w854]
                tunnel: w837 -> [w844 w855]
                tunnel: [w843 w855] -> w836
                tunnel: w831 -> [w842 _]
                tunnel: [w839 30] -> w817
                tunnel: w832 -> [w839 _]
                tunnel: [w838 w851] -> w821
                tunnel: w820 -> [w838 _]
                frame False {
                  n115 = String To Byte Array(string=w842) -> (unsigned byte array=w841:u8[])
                  n116 = Insert Into Array(array=w844, index=w840, new element=w841) -> (w843:dbl[])
                  n117 = Add(x=w840, y=1) -> (x+y=w846:i32)
                }
                frame True {
                  # "Go to read5P"
                  n118 = Byte Array To String(unsigned byte array=w855) -> (string=w856:string)
                  n119 = String Subset(string=w856, offset (0)=0, length (rest)=w854) -> (substring=w853:string)
                  n120 = Fract/Exp String To Number(string=w853) -> (number=w850:dbl)  [unwired: 3 in, 1 out]
                  n121 = Multiply(x=w850, y="Servo 4 Position Slope") -> (x*y=w852:dbl)
                  n122 = Add(x=w852, y="Servo 4 Position Intercept") -> (x+y=w851:dbl)
                  "Pos4 number" <- w851
                }
              }
            }
            frame "read5P" {
              n123 = Equal?(x=w890, y="v") -> (x = y?=w891:bool)
              n124 = case shown="True" w891 {
                tunnel: [w905 0] -> w888
                tunnel: w889 -> [w899 w912]
                tunnel: w895 -> [w903 w913]
                tunnel: [w902 w913] -> w894
                tunnel: w890 -> [w901 _]
                tunnel: [w898 36] -> w893
                tunnel: w892 -> [w898 _]
                tunnel: [w897 w907] -> w878
                tunnel: w876 -> [w897 _]
                frame False {
                  n125 = String To Byte Array(string=w901) -> (unsigned byte array=w900:u8[])
                  n126 = Insert Into Array(array=w903, index=w899, new element=w900) -> (w902:dbl[])
                  n127 = Add(x=w899, y=1) -> (x+y=w905:i32)
                }
                frame True {
                  # "Go to read1T"
                  n128 = Byte Array To String(unsigned byte array=w913) -> (string=w914:string)
                  n129 = String Subset(string=w914, offset (0)=0, length (rest)=w912) -> (substring=w911:string)
                  n130 = Fract/Exp String To Number(string=w911) -> (number=w909:dbl)  [unwired: 3 in, 1 out]
                  n131 = Multiply(x=w909, y="Servo 5 Position Slope") -> (x*y=w910:dbl)
                  n132 = Add(x=w910, y="Servo 5 Position Intercept") -> (x+y=w907:dbl)
                  "Pos5 number" <- w907
                }
              }
            }
            frame "read1T" {
              n133 = Equal?(x=w951, y="w") -> (x = y?=w952:bool)
              n134 = case shown="True" w952 {
                tunnel: [w964 0] -> w933
                tunnel: w934 -> [w958 w970]
                tunnel: w937 -> [w962 w972]
                tunnel: [w961 w972] -> w936
                tunnel: w951 -> [w960 _]
                tunnel: [w957 42] -> w954
                tunnel: w953 -> [w957 _]
                tunnel: [w956 w967] -> w930
                tunnel: w932 -> [w956 _]
                frame False {
                  n135 = String To Byte Array(string=w960) -> (unsigned byte array=w959:u8[])
                  n136 = Insert Into Array(array=w962, index=w958, new element=w959) -> (w961:dbl[])
                  n137 = Add(x=w958, y=1) -> (x+y=w964:i32)
                }
                frame True {
                  # "Go to read2T"
                  n138 = Byte Array To String(unsigned byte array=w972) -> (string=w973:string)
                  n139 = String Subset(string=w973, offset (0)=0, length (rest)=w970) -> (substring=w971:string)
                  n140 = Fract/Exp String To Number(string=w971) -> (number=w968:dbl)  [unwired: 3 in, 1 out]
                  n141 = Multiply(x=w968, y="Servo 1 Torque Slope") -> (x*y=w969:dbl)
                  n142 = Add(x=w969, y="Servo 1 Torque Intercept") -> (x+y=w967:dbl)
                  "Torq1 number" <- w967
                }
              }
            }
            frame "read2T" {
              n143 = Equal?(x=w1010, y="x") -> (x = y?=w1011:bool)
              n144 = case shown="True" w1011 {
                tunnel: [w1023 0] -> w985
                tunnel: w984 -> [w1017 w1029]
                tunnel: w996 -> [w1021 w1031]
                tunnel: [w1020 w1031] -> w995
                tunnel: w1010 -> [w1019 _]
                tunnel: [w1016 48] -> w1013
                tunnel: w1012 -> [w1016 _]
                tunnel: [w1015 w1026] -> w980
                tunnel: w983 -> [w1015 _]
                frame False {
                  n145 = String To Byte Array(string=w1019) -> (unsigned byte array=w1018:u8[])
                  n146 = Insert Into Array(array=w1021, index=w1017, new element=w1018) -> (w1020:dbl[])
                  n147 = Add(x=w1017, y=1) -> (x+y=w1023:i32)
                }
                frame True {
                  # "Go to read3T"
                  n148 = Byte Array To String(unsigned byte array=w1031) -> (string=w1032:string)
                  n149 = String Subset(string=w1032, offset (0)=0, length (rest)=w1029) -> (substring=w1030:string)
                  n150 = Fract/Exp String To Number(string=w1030) -> (number=w1027:dbl)  [unwired: 3 in, 1 out]
                  n151 = Multiply(x=w1027, y="Servo 2 Torque Slope") -> (x*y=w1028:dbl)
                  n152 = Add(x=w1028, y="Servo 2 Torque Intercept") -> (x+y=w1026:dbl)
                  "Torq2 number" <- w1026
                }
              }
            }
            frame "read3T" {
              n153 = Equal?(x=w1069, y="y") -> (x = y?=w1070:bool)
              n154 = case shown="True" w1070 {
                tunnel: [w1082 0] -> w1045
                tunnel: w1044 -> [w1076 w1088]
                tunnel: w1048 -> [w1080 w1090]
                tunnel: [w1079 w1090] -> w1047
                tunnel: w1069 -> [w1078 _]
                tunnel: [w1075 54] -> w1072
                tunnel: w1071 -> [w1075 _]
                tunnel: [w1074 w1086] -> w1051
                tunnel: w1056 -> [w1074 _]
                frame False {
                  n155 = String To Byte Array(string=w1078) -> (unsigned byte array=w1077:u8[])
                  n156 = Insert Into Array(array=w1080, index=w1076, new element=w1077) -> (w1079:dbl[])
                  n157 = Add(x=w1076, y=1) -> (x+y=w1082:i32)
                }
                frame True {
                  # "Go to read4T"
                  n158 = Byte Array To String(unsigned byte array=w1090) -> (string=w1091:string)
                  n159 = String Subset(string=w1091, offset (0)=0, length (rest)=w1088) -> (substring=w1089:string)
                  n160 = Fract/Exp String To Number(string=w1089) -> (number=w1085:dbl)  [unwired: 3 in, 1 out]
                  n161 = Multiply(x=w1085, y="Servo 3 Torque Slope") -> (x*y=w1087:dbl)
                  n162 = Add(x=w1087, y="Servo 3 Torque Intercept") -> (x+y=w1086:dbl)
                  "Torq3 number" <- w1086
                }
              }
            }
            frame "read4T" {
              n163 = Equal?(x=w1128, y="z") -> (x = y?=w1129:bool)
              n164 = case shown="True" w1129 {
                tunnel: [w1141 0] -> w1101
                tunnel: w1100 -> [w1135 w1147]
                tunnel: w1106 -> [w1139 w1149]
                tunnel: [w1138 w1149] -> w1107
                tunnel: w1128 -> [w1137 _]
                tunnel: [w1134 60] -> w1131
                tunnel: w1130 -> [w1134 _]
                tunnel: [w1133 w1144] -> w1110
                tunnel: w1114 -> [w1133 _]
                frame False {
                  n165 = String To Byte Array(string=w1137) -> (unsigned byte array=w1136:u8[])
                  n166 = Insert Into Array(array=w1139, index=w1135, new element=w1136) -> (w1138:dbl[])
                  n167 = Add(x=w1135, y=1) -> (x+y=w1141:i32)
                }
                frame True {
                  # "Go to read5T"
                  n168 = Byte Array To String(unsigned byte array=w1149) -> (string=w1150:string)
                  n169 = String Subset(string=w1150, offset (0)=0, length (rest)=w1147) -> (substring=w1148:string)
                  n170 = Fract/Exp String To Number(string=w1148) -> (number=w1145:dbl)  [unwired: 3 in, 1 out]
                  n171 = Multiply(x=w1145, y="Servo 4 Torque Slope") -> (x*y=w1146:dbl)
                  n172 = Add(x=w1146, y="Servo 4 Torque Intercept") -> (x+y=w1144:dbl)
                  "Torq4 number" <- w1144
                }
              }
            }
            frame "read5T" {
              n173 = Equal?(x=w1187, y="!") -> (x = y?=w1188:bool)
              n174 = case shown="True" w1188 {
                tunnel: [w1200 0] -> w1163
                tunnel: w1162 -> [w1194 w1206]
                tunnel: w1165 -> [w1198 w1208]
                tunnel: [w1197 w1208] -> w1166
                tunnel: w1187 -> [w1196 _]
                tunnel: [w1193 0] -> w1190
                tunnel: w1189 -> [w1193 _]
                tunnel: [w1192 w1201] -> w1172
                tunnel: w1173 -> [w1192 _]
                frame False {
                  n175 = String To Byte Array(string=w1196) -> (unsigned byte array=w1195:u8[])
                  n176 = Insert Into Array(array=w1198, index=w1194, new element=w1195) -> (w1197:dbl[])
                  n177 = Add(x=w1194, y=1) -> (x+y=w1200:i32)
                }
                frame True {
                  # "Go to none11"
                  n178 = Byte Array To String(unsigned byte array=w1208) -> (string=w1209:string)
                  n179 = String Subset(string=w1209, offset (0)=0, length (rest)=w1206) -> (substring=w1207:string)
                  n180 = Fract/Exp String To Number(string=w1207) -> (number=w1204:dbl)  [unwired: 3 in, 1 out]
                  n181 = Multiply(x=w1204, y="Servo 5 Torque Slope") -> (x*y=w1205:dbl)
                  n182 = Add(x=w1205, y="Servo 5 Torque Intercept") -> (x+y=w1201:dbl)
                  "Torq5 number" <- w1201
                }
              }
            }
          }
        }
      }
    }
    n183 = call-poly <vilib>:"Mean.vi"("X"=w87) -> ("mean"=w57:dbl)  [unwired: 1 out]
    "Calculated Time Delay" <- w57
    n184 = Bundle(0, "mean"=w57, w375) -> (→"Bytes at port":cluster{i32, "mean":dbl, dbl[]})  [unwired: 1 in]
    n185 = Subtract(x=w59, y=1) -> (x-y=w318:i32)
    n186 = Subtract(x=w59, y=1) -> (x-y=w307:i32)
    n187 = Subtract(x=w59, y=1) -> (x-y=w310:i32)
    n188 = Subtract(x=w59, y=1) -> (x-y=w301:i32)
    n189 = Subtract(x=w59, y=1) -> (x-y=w304:i32)
    n190 = Index Array(array=w305, index=w307) -> (element=w289:dbl)
    n191 = Index Array(array=w308, index=w310) -> (element=w294:dbl)
    n192 = Index Array(array=w302, index=w304) -> (element=w283:dbl)
    n193 = Index Array(array=w272, index=w301) -> (element=w274:dbl)
    n194 = Index Array(array=w316, index=w318) -> (element=w313:dbl)
    n195 = Less?(x=w277, y="Lowest Servo Angle") -> (x < y?=w278:bool)
    n196 = Greater?(x=w277, y="Highest Servo Angle") -> (0:w280:bool)
    n197 = Or(x=w280, y=w278) -> (x .or. y?=w279:bool)
    n198 = case shown="True" w279 {
      tunnel: w274 -> [_ w452]
      tunnel: w277 -> [w450 _]
      tunnel: [w450 w452] -> w273
      tunnel: [FALSE TRUE] -> w215
      frame False {
      }
      frame True {
      }
    }
    n199 = Greater?(x=w281, y="Highest Servo Angle") -> (0:w284:bool)
    n200 = Less?(x=w281, y="Lowest Servo Angle") -> (x < y?=w285:bool)
    n201 = Or(x=w284, y=w285) -> (x .or. y?=w286:bool)
    n202 = case shown="True" w286 {
      tunnel: w283 -> [_ w456]
      tunnel: w281 -> [w454 _]
      tunnel: [w454 w456] -> w282
      tunnel: [FALSE TRUE] -> w216
      frame False {
      }
      frame True {
      }
    }
    n203 = Or(x=w216, y=w215) -> (x .or. y?=w213:bool)
    n204 = Greater?(x=w287, y="Highest Servo Angle") -> (0:w292:bool)
    n205 = Less?(x=w287, y="Lowest Servo Angle") -> (x < y?=w290:bool)
    n206 = Or(x=w292, y=w290) -> (x .or. y?=w291:bool)
    n207 = Tick Count (ms)() -> (millisecond timer value=w133:u32)
    n208 = case shown="True" w291 {
      tunnel: w289 -> [_ w460]
      tunnel: w287 -> [w458 _]
      tunnel: [w458 w460] -> w288
      tunnel: [FALSE TRUE] -> w214
      frame False {
      }
      frame True {
      }
    }
    n209 = Divide(x=w133, y=1000) -> (x/y=w131:dbl)
    n210 = Or(x=w214, y=w213) -> (x .or. y?=w211:bool)
    n211 = Sine(x=w131) -> (sin(x)=w122:dbl)
    n212 = Greater?(x=w293, y="Highest Servo Angle") -> (0:w298:bool)
    n213 = Less?(x=w293, y="Lowest Servo Angle") -> (x < y?=w296:bool)
    n214 = Or(x=w298, y=w296) -> (x .or. y?=w297:bool)
    n215 = case shown="True" w297 {
      tunnel: w294 -> [_ w464]
      tunnel: w293 -> [w462 _]
      tunnel: [w462 w464] -> w295
      tunnel: [FALSE TRUE] -> w212
      frame False {
      }
      frame True {
      }
    }
    n216 = Multiply(x=2, y=w122) -> (x*y=w124:dbl)
    n217 = Or(x=w212, y=w211) -> (x .or. y?=w209:bool)
    n218 = Multiply(x=w122, y=0.1) -> (x*y=w123:dbl)
    n219 = Less?(x=w311, y="Lowest Servo Angle") -> (x < y?=w312:bool)
    n220 = Greater?(x=w311, y="Highest Servo Angle") -> (0:w315:bool)
    n221 = Or(x=w315, y=w312) -> (x .or. y?=w314:bool)
    n222 = Insert Into Array(array=w126, index=w59, new element=w124) -> (w65:dbl[])
    n223 = Insert Into Array(array=w125, index=w59, new element=w123) -> (w64:dbl[])
    n224 = Insert Into Array(array=w127, index=w59, new element=w122) -> (w66:dbl[])
    n225 = case shown="True" w314 {
      tunnel: w313 -> [_ w468]
      tunnel: w311 -> [w466 _]
      tunnel: [w466 w468] -> w299
      tunnel: [FALSE TRUE] -> w210
      frame False {
      }
      frame True {
      }
    }
    n226 = Or(x=w210, y=w209) -> (x .or. y?=→"Minimum or Maximum Angle Exceeded":bool)
    n227 = call <vilib>:"Amplitude and Phase Spectrum.vi"("dt"=w57, "Signal (V)"=w66) -> ("df"=w118:dbl, "Amp Spectrum Mag (Vrms)"=w119:dbl[])  [unwired: 1 in, 1 out]
    n228 = Insert Into Array(array=w316, index=w59, new element=w299) -> (w69:dbl[])
    n229 = Insert Into Array(array=w308, index=w59, new element=w295) -> (w71:dbl[])
    n230 = Insert Into Array(array=w272, index=w59, new element=w273) -> (w85:dbl[])
    n231 = Insert Into Array(array=w305, index=w59, new element=w288) -> (w75:dbl[])
    n232 = Insert Into Array(array=w302, index=w59, new element=w282) -> (w79:dbl[])
    n233 = Greater?(x=w194, y="Max Torque") -> (0:w188:bool)
    n234 = Bundle("timeout (s)"=0.0, "df"=w118, "Amp Spectrum Mag (Vrms)"=w119) -> (→"Lift FFT":T3)  [unwired: 1 in]
    n235 = Greater?(x=w190, y="Max Torque") -> (0:w187:bool)
    n236 = Greater?(x=w191, y="Max Torque") -> (0:w186:bool)
    n237 = Or(x=w187, y=w188) -> (x .or. y?=w185:bool)
    n238 = Greater?(x=w192, y="Max Torque") -> (0:w184:bool)
    n239 = Or(x=w186, y=w185) -> (x .or. y?=w181:bool)
    n240 = Greater?(x=w193, y="Max Torque") -> (0:w183:bool)
    n241 = Or(x=w184, y=w181) -> (x .or. y?=w182:bool)
    n242 = Bundle(w113, 20, 0.5, 0.1, w113) -> (w117:cluster{i32, i32, dbl, dbl, i32})  [unwired: 1 in]
    n243 = Subtract(x=w162, y=w166) -> (x-y=w167:dbl)
    n244 = Bundle(w109, 1, 0.1, 0.05, w109) -> (w108:cluster{i32, i32, dbl, dbl, i32})  [unwired: 1 in]
    n245 = Insert Into Array(array=w327, index=w59, new element=w194) -> (w207:dbl[])
    n246 = Insert Into Array(array=w326, index=w59, new element=w190) -> (w205:dbl[])
    n247 = Insert Into Array(array=w323, index=w59, new element=w193) -> (w206:dbl[])
    n248 = Or(x=w183, y=w182) -> (x .or. y?=→"Maximum Torque Exceeded":bool)
    n249 = Insert Into Array(array=w325, index=w59, new element=w191) -> (w204:dbl[])
    n250 = Subtract(x=w163, y=w166) -> (x-y=w168:dbl)
    n251 = Insert Into Array(array=w324, index=w59, new element=w192) -> (w203:dbl[])
    n252 = Subtract(x=w161, y=w166) -> (x-y=w169:dbl)
    n253 = property on="Lift FFT" class="WFGraph (strict)"("XScale.Range"=w117) -> ()  [unwired: 2 in, 2 out]
    n254 = Subtract(x=w164, y=w166) -> (x-y=w170:dbl)
    n255 = Subtract(x=w165, y=w166) -> (x-y=w171:dbl)
    n256 = property on="Lift FFT" class="WFGraph (strict)"("YScale.Range"=w108) -> ()  [unwired: 2 in, 2 out]
    n257 = Build Array(w171, w170, w169, w168, w167) -> (w136:dbl[])
    "Output Angles" <- w136
    n258 = call "PlotSubArray.vi"("Time Step (s)"=w57, "Plot Last x Seconds"="Plot Last x Seconds", "Iteration"=w59, "Array"=w79) -> ("Sub Array"=w50:dbl[], "Time Offset"=w77:dbl)  [unwired: 6 in]
    n259 = call "PlotSubArray.vi"("Time Step (s)"=w57, "Plot Last x Seconds"="Plot Last x Seconds", "Iteration"=w59, "Array"=w70) -> ("Sub Array"=w56:dbl[])  [unwired: 6 in, 1 out]
    n260 = call "PlotSubArray.vi"("Time Step (s)"=w57, "Plot Last x Seconds"="Plot Last x Seconds", "Iteration"=w59, "Array"=w78) -> ("Sub Array"=w49:dbl[])  [unwired: 6 in, 1 out]
    n261 = call "PlotSubArray.vi"("Time Step (s)"=w57, "Plot Last x Seconds"="Plot Last x Seconds", "Iteration"=w59, "Array"=w71) -> ("Sub Array"=w54:dbl[], "Time Offset"=w73:dbl)  [unwired: 6 in]
    n262 = call "PlotSubArray.vi"("Time Step (s)"=w57, "Plot Last x Seconds"="Plot Last x Seconds", "Iteration"=w59, "Array"=w72) -> ("Sub Array"=w53:dbl[])  [unwired: 6 in, 1 out]
    n263 = call "PlotSubArray.vi"("Time Step (s)"=w57, "Plot Last x Seconds"="Plot Last x Seconds", "Iteration"=w59, "Array"=w76) -> ("Sub Array"=w52:dbl[])  [unwired: 6 in, 1 out]
    n264 = call "PlotSubArray.vi"("Time Step (s)"=w57, "Plot Last x Seconds"="Plot Last x Seconds", "Iteration"=w59, "Array"=w75) -> ("Sub Array"=w51:dbl[], "Time Offset"=w74:dbl)  [unwired: 6 in]
    n265 = call "PlotSubArray.vi"("Time Step (s)"=w57, "Plot Last x Seconds"="Plot Last x Seconds", "Iteration"=w59, "Array"=w86) -> ("Sub Array"=w47:dbl[])  [unwired: 6 in, 1 out]
    n266 = call "PlotSubArray.vi"("Time Step (s)"=w57, "Plot Last x Seconds"="Plot Last x Seconds", "Iteration"=w59, "Array"=w85) -> ("Sub Array"=w48:dbl[], "Time Offset"=w84:dbl)  [unwired: 6 in]
    n267 = call "PlotSubArray.vi"("Time Step (s)"=w57, "Plot Last x Seconds"="Plot Last x Seconds", "Iteration"=w59, "Array"=w69) -> ("Sub Array"=w55:dbl[], "Time Offset"=w68:dbl)  [unwired: 6 in]
    n268 = Divide(x="Length of Segments", y=100) -> (x/y=w147:dbl)
    n269 = Initialize Array(0.0 ("element"), 1 ("dimension size")) -> (w174:dbl[])
    n270 = Initialize Array(0.0 ("element"), 1 ("dimension size")) -> (w173:dbl[])
    n271 = Build Array(w52, w51) -> (w342:dbl[][])
    n272 = Build Array(w47, w48) -> (w83:dbl[][])
    n273 = Build Array(w49, w50) -> (w81:dbl[][])
    n274 = Build Array(w56, w55) -> (w344:dbl[][])
    n275 = call "PlotSubArray.vi"("Time Step (s)"=w57, "Plot Last x Seconds"="Plot Last x Seconds", "Iteration"=w59, "Array"=w207) -> ("Sub Array"=w201:dbl[], "Time Offset"=w202:dbl)  [unwired: 6 in]
    n276 = Build Array(w53, w54) -> (w343:dbl[][])
    n277 = call "PlotSubArray.vi"("Time Step (s)"=w57, "Plot Last x Seconds"="Plot Last x Seconds", "Iteration"=w59, "Array"=w205) -> ("Sub Array"=w200:dbl[])  [unwired: 6 in, 1 out]
    n278 = call "PlotSubArray.vi"("Time Step (s)"=w57, "Plot Last x Seconds"="Plot Last x Seconds", "Iteration"=w59, "Array"=w204) -> ("Sub Array"=w199:dbl[])  [unwired: 6 in, 1 out]
    n279 = call "PlotSubArray.vi"("Time Step (s)"=w57, "Plot Last x Seconds"="Plot Last x Seconds", "Iteration"=w59, "Array"=w203) -> ("Sub Array"=w198:dbl[])  [unwired: 6 in, 1 out]
    n280 = call "PlotSubArray.vi"("Time Step (s)"=w57, "Plot Last x Seconds"="Plot Last x Seconds", "Iteration"=w59, "Array"=w206) -> ("Sub Array"=w197:dbl[])  [unwired: 6 in, 1 out]
    n281 = Bundle("Time Offset"=w77, "mean"=w57, w81) -> (→"Servo 4 Position":cluster{" Time Offset":dbl, "mean":dbl, dbl[][]})  [unwired: 1 in]
    n282 = Bundle("Time Offset"=w74, "mean"=w57, w342) -> (→"Servo 3 Position":cluster{" Time Offset":dbl, "mean":dbl, dbl[][]})  [unwired: 1 in]
    n283 = Bundle("Time Offset"=w73, "mean"=w57, w343) -> (→"Servo 2 Position":cluster{" Time Offset":dbl, "mean":dbl, dbl[][]})  [unwired: 1 in]
    n284 = Bundle("Time Offset"=w84, "mean"=w57, w83) -> (→"Servo 5 Position":cluster{" Time Offset":dbl, "mean":dbl, dbl[][]})  [unwired: 1 in]
    n285 = Bundle("Time Offset"=w68, "mean"=w57, w344) -> (→"Servo 1 Position":cluster{" Time Offset":dbl, "mean":dbl, dbl[][]})  [unwired: 1 in]
    n286 = Build Array(w201, w200, w199, w198, w197) -> (w196:dbl[][])
    n287 = for {
      N: w92 -> [_]
      shift-right: [w388] -> _
      shift-left: 0.0 -> [w405]
      tunnel: w136 -> [w404]
      shift-right: [w398] -> w143
      shift-left: w174 -> [w386]
      shift-right: [w397] -> w142
      shift-left: w173 -> [w385]
      tunnel: w147 -> [w384]
      i -> [w396]
      (unwired) 100
      # "phi"
      # "L"
      n288 = Index Array(array=w404, index=w396) -> (element=w403:dbl)
      n289 = Index Array(array=w386, index=w396) -> (element=w402:dbl)
      n290 = Index Array(array=w385, index=w396) -> (element=w399:dbl)
      n291 = Divide(x=3.141592653589793, y=180) -> (x/y=w387:dbl)
      n292 = Add(x=w403, y=w405) -> (x+y=w388:dbl)
      n293 = Multiply(x=w387, y=w388) -> (x*y=w390:dbl)
      n294 = Multiply(x=w387, y=w388) -> (x*y=w389:dbl)
      n295 = Increment(x=w396) -> (x+1=w395:i32)
      n296 = Cosine(x=w390) -> (cos(x)=w394:dbl)
      n297 = Sine(x=w389) -> (sin(x)=w393:dbl)
      n298 = Multiply(x=w394, y=w384) -> (x*y=w401:dbl)
      n299 = Multiply(x=w384, y=w393) -> (x*y=w400:dbl)
      n300 = Add(x=w402, y=w401) -> (x+y=w383:dbl)
      n301 = Add(x=w400, y=w399) -> (x+y=w382:dbl)
      n302 = Insert Into Array(array=w386, index=w395, new element=w383) -> (w398:dbl[])
      n303 = Insert Into Array(array=w385, index=w395, new element=w382) -> (w397:dbl[])
    }
    n304 = Bundle("Time Offset"=w202, "mean"=w57, w196) -> (→"Servo Torque":cluster{" Time Offset":dbl, "mean":dbl, dbl[][]})  [unwired: 1 in]
    n305 = call "PlotSubArray.vi"("Time Step (s)"=w57, "Plot Last x Seconds"="Plot Last x Seconds", "Iteration"=w59, "Array"=w66) -> ("Sub Array"=w63:dbl[], "Time Offset"=w60:dbl)  [unwired: 6 in]
    n306 = call "PlotSubArray.vi"("Time Step (s)"=w57, "Plot Last x Seconds"="Plot Last x Seconds", "Iteration"=w59, "Array"=w65) -> ("Sub Array"=w62:dbl[])  [unwired: 6 in, 1 out]
    n307 = call "PlotSubArray.vi"("Time Step (s)"=w57, "Plot Last x Seconds"="Plot Last x Seconds", "Iteration"=w59, "Array"=w64) -> ("Sub Array"=w61:dbl[])  [unwired: 6 in, 1 out]
    n308 = Increment(x=w92) -> (x+1=w160:dbl)
    n309 = Increment(x=w92) -> (x+1=w157:dbl)
    n310 = Increment(x=w92) -> (x+1=w144:dbl)
    n311 = Multiply(x=w160, y="Length of Segments") -> (x*y=w158:dbl)
    n312 = Multiply(x=w157, y="Length of Segments") -> (x*y=w154:dbl)
    n313 = Divide(x="Length of Segments", y=5) -> (x/y=w155:dbl)
    n314 = Divide(x="Length of Segments", y=5) -> (x/y=w156:dbl)
    n315 = Multiply(x=-1, y=w158) -> (x*y=w159:dbl)
    n316 = Build Array(w63, w62, w61) -> (w128:dbl[][])
    n317 = Bundle(w150, w154, w147, w155, w150) -> (w149:cluster{i32, dbl, dbl, dbl, i32})  [unwired: 1 in]
    n318 = for {
      N: w144 -> [_]
      tunnel: w143 -> [w381] mode=indexing
      tunnel: w142 -> [w379] mode=indexing
      tunnel: [w378] -> w140 mode=indexing
      tunnel: [w377] -> w139 mode=indexing
      w380 = 100
      # "Convert nodes from m to cm"
      n319 = Multiply(x=w381, y=w380) -> (x*y=w378:dbl)
      n320 = Multiply(x=w380, y=w379) -> (x*y=w377:dbl)
    }
    n321 = Bundle(w159, w158, w147, w156, w159) -> (w148:cluster{dbl, dbl, dbl, dbl, dbl})  [unwired: 1 in]
    n322 = Bundle("Time Offset"=w60, "mean"=w57, w128) -> (→"Force and Moment Data":cluster{" Time Offset":dbl, "mean":dbl, dbl[][]})  [unwired: 1 in]
    n323 = property on="Waveform" class="XYGraph (strict)"("XScale.Range"=w149) -> ()  [unwired: 2 in, 2 out]
    n324 = property on="Waveform" class="XYGraph (strict)"("YScale.Range"=w148) -> ()  [unwired: 2 in, 2 out]
    n325 = property on="Waveform" class="XYGraph (strict)"("Plot.Point Style"=u8 2) -> ()  [unwired: 2 in, 2 out]
    n326 = Bundle(w140, w139) -> (w138:cluster{dbl[], dbl[]})  [unwired: 1 in]
    n327 = Build Array(w145, w138) -> (→"Waveform":cluster{"X Nodes":dbl[], "Y Nodes":dbl[]}[])
  }
  n328 = VISA Close(VISA resource name=w33, error in (no error)=w32) -> ()  [unwired: 1 out]
  n329 = case shown="True" w34 {
    tunnel: w35 -> [_ w1287]
    tunnel: w31 -> [_ w1286]
    tunnel: w27 -> [_ w1275]
    tunnel: w26 -> [_ w1274]
    tunnel: w25 -> [_ w1273]
    tunnel: w24 -> [_ w1264]
    tunnel: w23 -> [_ w1263]
    tunnel: w22 -> [_ w1262]
    tunnel: w21 -> [_ w1261]
    tunnel: w20 -> [_ w1252]
    tunnel: w19 -> [_ w1251]
    tunnel: w18 -> [_ w1250]
    tunnel: w17 -> [_ w1249]
    tunnel: w16 -> [_ w1247]
    tunnel: w15 -> [_ w1237]
    tunnel: w14 -> [_ w1236]
    tunnel: w13 -> [_ w1235]
    tunnel: w12 -> [_ w1234]
    frame False {
    }
    frame True {
      n330 = call "Convert to Dynamic Data9"("Array"=w1261) -> ("Dynamic Data Type"=w1266:dynamicdata)  [unwired: 3 in]
      n331 = call "Convert to Dynamic Data11"("Array"=w1251) -> ("Dynamic Data Type"=w1258:dynamicdata)  [unwired: 3 in]
      n332 = call "Convert to Dynamic Data13"("Array"=w1249) -> ("Dynamic Data Type"=w1254:dynamicdata)  [unwired: 3 in]
      n333 = call "Convert to Dynamic Data"("Array"=w1286) -> ("Dynamic Data Type"=w1285:dynamicdata)  [unwired: 3 in]
      n334 = call "Convert to Dynamic Data12"("Array"=w1250) -> ("Dynamic Data Type"=w1256:dynamicdata)  [unwired: 3 in]
      n335 = call "Convert to Dynamic Data10"("Array"=w1252) -> ("Dynamic Data Type"=w1260:dynamicdata)  [unwired: 3 in]
      n336 = call "Convert to Dynamic Data17"("Array"=w1235) -> ("Dynamic Data Type"=w1240:dynamicdata)  [unwired: 3 in]
      n337 = call "Convert to Dynamic Data18"("Array"=w1234) -> ("Dynamic Data Type"=w1238:dynamicdata)  [unwired: 3 in]
      n338 = call "Convert to Dynamic Data16"("Array"=w1236) -> ("Dynamic Data Type"=w1242:dynamicdata)  [unwired: 3 in]
      n339 = call "Convert to Dynamic Data15"("Array"=w1237) -> ("Dynamic Data Type"=w1244:dynamicdata)  [unwired: 3 in]
      n340 = call "Convert to Dynamic Data14"("Array"=w1247) -> ("Dynamic Data Type"=w1246:dynamicdata)  [unwired: 3 in]
      n341 = call "Convert to Dynamic Data2"("Array"=w1287) -> ("Dynamic Data Type"=w1284:dynamicdata)  [unwired: 3 in]
      n342 = call "Convert to Dynamic Data6"("Array"=w1264) -> ("Dynamic Data Type"=w1272:dynamicdata)  [unwired: 3 in]
      n343 = call "Convert to Dynamic Data8"("Array"=w1262) -> ("Dynamic Data Type"=w1268:dynamicdata)  [unwired: 3 in]
      n344 = call "Convert to Dynamic Data7"("Array"=w1263) -> ("Dynamic Data Type"=w1270:dynamicdata)  [unwired: 3 in]
      n345 = call "Convert to Dynamic Data5"("Array"=w1275) -> ("Dynamic Data Type"=w1280:dynamicdata)  [unwired: 3 in]
      n346 = call "Convert to Dynamic Data4"("Array"=w1274) -> ("Dynamic Data Type"=w1279:dynamicdata)  [unwired: 3 in]
      n347 = call "Convert to Dynamic Data3"("Array"=w1273) -> ("Dynamic Data Type"=w1281:dynamicdata)  [unwired: 3 in]
      n348 = xnode "Set Dynamic Data Attributes"("Signals In"=w1279, "Signal Name"="Lift Force") -> ("Signals Out"=w1232:dynamicdata)  [unwired: 2 in, 1 out]
      n349 = xnode "Set Dynamic Data Attributes"("Signals In"=w1280, "Signal Name"="Drag Force") -> ("Signals Out"=w1233:dynamicdata)  [unwired: 2 in, 1 out]
      n350 = xnode "Set Dynamic Data Attributes"("Signals In"=w1281, "Signal Name"="Yaw Moment") -> ("Signals Out"=w1231:dynamicdata)  [unwired: 2 in, 1 out]
      n351 = xnode "Set Dynamic Data Attributes"("Signals In"=w1284, "Signal Name"="Servo 1 Commanded Position") -> ("Signals Out"=w1230:dynamicdata)  [unwired: 2 in, 1 out]
      n352 = xnode "Set Dynamic Data Attributes"("Signals In"=w1272, "Signal Name"="Servo 2 Commanded Position") -> ("Signals Out"=w1229:dynamicdata)  [unwired: 2 in, 1 out]
      n353 = xnode "Set Dynamic Data Attributes"("Signals In"=w1268, "Signal Name"="Servo 4 Commanded Position") -> ("Signals Out"=w1227:dynamicdata)  [unwired: 2 in, 1 out]
      n354 = xnode "Set Dynamic Data Attributes"("Signals In"=w1270, "Signal Name"="Servo 3 Commanded Position") -> ("Signals Out"=w1228:dynamicdata)  [unwired: 2 in, 1 out]
      n355 = xnode "Set Dynamic Data Attributes"("Signals In"=w1266, "Signal Name"="Servo 5 Commanded Position") -> ("Signals Out"=w1226:dynamicdata)  [unwired: 2 in, 1 out]
      n356 = xnode "Set Dynamic Data Attributes"("Signals In"=w1285, "Signal Name"="Servo 1 Feedback Position") -> ("Signals Out"=w1225:dynamicdata)  [unwired: 2 in, 1 out]
      n357 = xnode "Set Dynamic Data Attributes"("Signals In"=w1256, "Signal Name"="Servo 1 Feedback Position") -> ("Signals Out"=w1222:dynamicdata)  [unwired: 2 in, 1 out]
      n358 = xnode "Set Dynamic Data Attributes"("Signals In"=w1258, "Signal Name"="Servo 1 Feedback Position") -> ("Signals Out"=w1223:dynamicdata)  [unwired: 2 in, 1 out]
      n359 = xnode "Set Dynamic Data Attributes"("Signals In"=w1240, "Signal Name"="Servo 4  Torque") -> ("Signals Out"=w1217:dynamicdata)  [unwired: 2 in, 1 out]
      n360 = xnode "Set Dynamic Data Attributes"("Signals In"=w1238, "Signal Name"="Servo 5  Torque") -> ("Signals Out"=w1216:dynamicdata)  [unwired: 2 in, 1 out]
      n361 = xnode "Set Dynamic Data Attributes"("Signals In"=w1260, "Signal Name"="Servo 1 Feedback Position") -> ("Signals Out"=w1224:dynamicdata)  [unwired: 2 in, 1 out]
      n362 = xnode "Set Dynamic Data Attributes"("Signals In"=w1242, "Signal Name"="Servo 3  Torque") -> ("Signals Out"=w1218:dynamicdata)  [unwired: 2 in, 1 out]
      n363 = xnode "Set Dynamic Data Attributes"("Signals In"=w1254, "Signal Name"="Servo 1 Feedback Position") -> ("Signals Out"=w1221:dynamicdata)  [unwired: 2 in, 1 out]
      n364 = xnode "Set Dynamic Data Attributes"("Signals In"=w1244, "Signal Name"="Servo 2  Torque") -> ("Signals Out"=w1219:dynamicdata)  [unwired: 2 in, 1 out]
      n365 = xnode "Set Dynamic Data Attributes"("Signals In"=w1246, "Signal Name"="Servo 1  Torque") -> ("Signals Out"=w1220:dynamicdata)  [unwired: 2 in, 1 out]
      n366 = Merge Signals(w1233, w1232, w1231, w1230, w1229, w1228, w1227, w1226, w1225, w1224, w1223, w1222, w1221, w1220, w1219, w1218, w1217, w1216) -> (w1215:dynamicdata)
      n367 = call "Write To Measurement File"("Signals"=w1215, "Filename"="Filename", "Comment"="Comment") -> ()  [unwired: 14 in, 3 out]
    }
  }
